vi "Read XML_Extra Checks_Check Tx Channels Default Values Presence.vi"(8 "error in (no error)":errorcluster, 11 "Channels In":T1[](array[typedef])) -> (0 "error out":errorcluster)   [LabVIEW 2016]
doc: "This VI checks that for a given Hardware Channel, all parameters have a unique combination of Parameter settings: Hardware Channel, Label Decimal and Parameter Name. If there are multiple duplicates, the function returns all duplicates."
uses:
  XML_Channel.ctl
  XML_Label.ctl
  XML_Parameter.ctl
  <userlib>/_OpenG.lib/array/array.llb/Filter 1D Array with Scalar (Boolean)__ogtk.vi
panel:
  out "Error Source":string
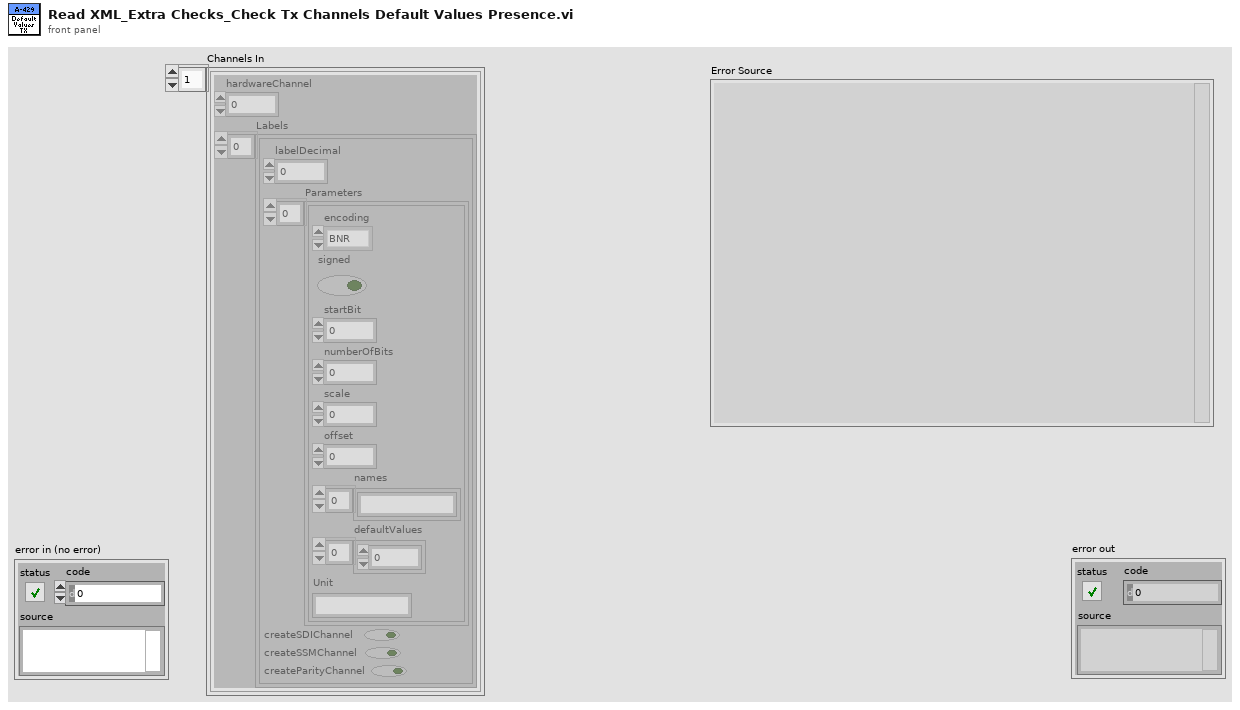
[diagram p1: front panel]
types:
  T1 = typedef "XML_Channel.ctl" = cluster{"hardwareChannel":i32, "Labels":T2[]}
  T2 = typedef "XML_Label.ctl" = cluster{"labelDecimal":i32, "Parameters":T3[], "createSDIChannel":bool, "createSSMChannel":bool, "createParityChannel":bool}
  T3 = typedef "XML_Parameter.ctl" = cluster{"encoding":enum16{"BNR", "BCD", "Discrete"}, "signed":bool, "startBit":i32, "numberOfBits":i32, "scale":dbl, "offset":dbl, "names":string[], "defaultValues":dbl[], "Unit":string}
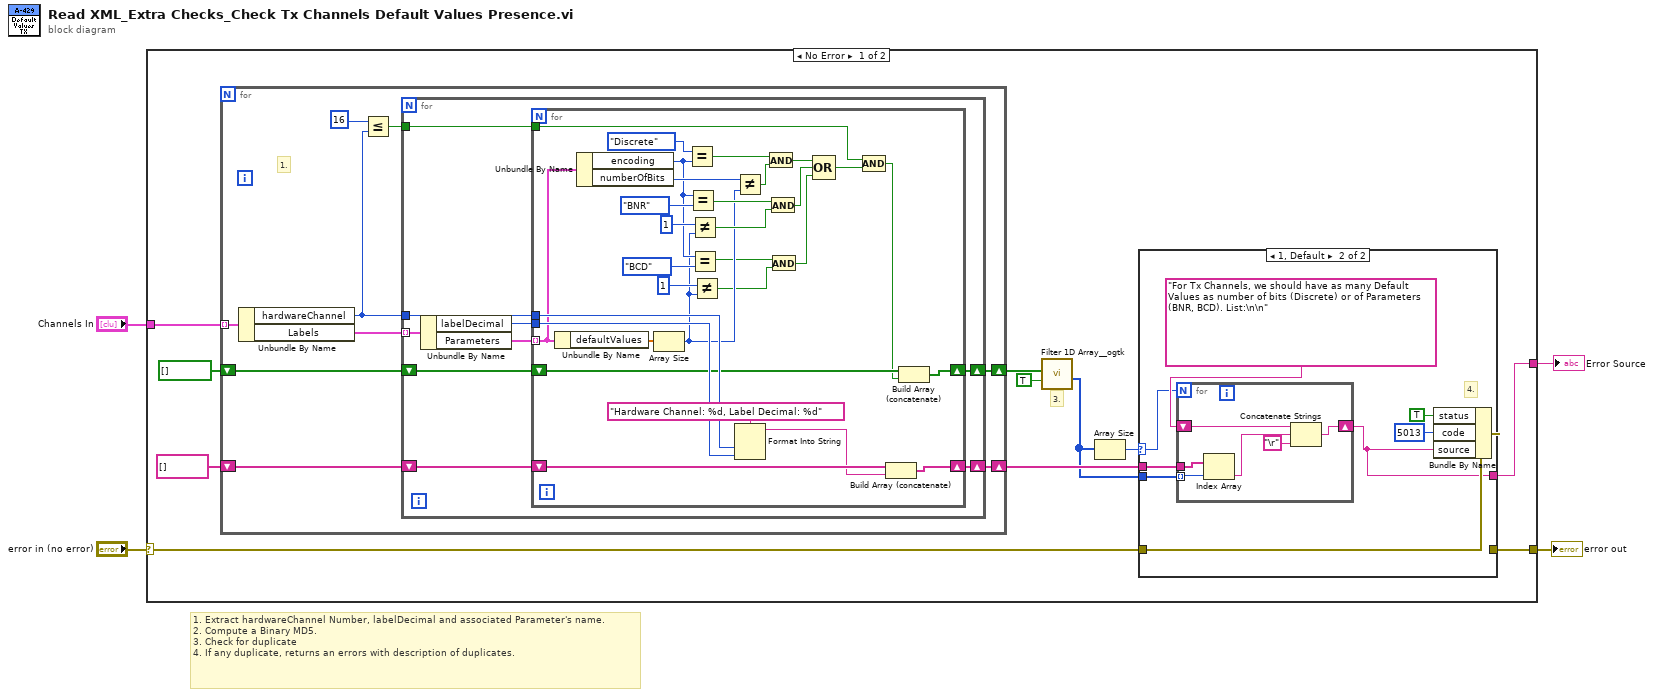
[diagram p0: block diagram]
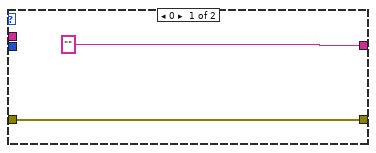
[diagram p2: hidden frame]
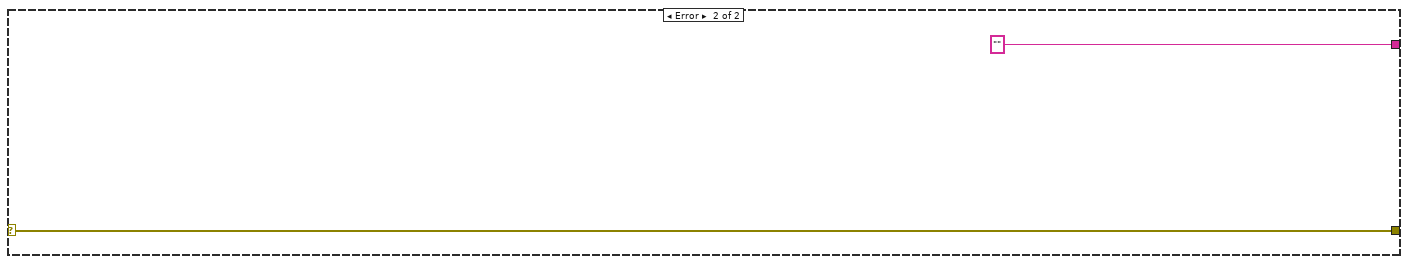
[diagram p3: hidden frame]
diagram:
  # "1. Extract hardwareChannel Number, labelDecimal and associated Parameter's name.\n2. Compute a Binary MD5.\n3. Check for duplicate\n4. If any duplicate, returns an errors with description of duplicates."
  n1 = case shown="No Error" "error in (no error)" {
    selector: "error in (no error)" -> [w14 w82]
    tunnel: [w12 w82] -> w3
    tunnel: "Channels In" -> [w13 _]
    tunnel: [w11 ""] -> w1
    frame No Error {
      # "3."
      n2 = for {
        tunnel: w13 -> [w41] mode=indexing
        shift-right: [w38] -> w8
        shift-left: bool[] [] -> [w39]
        shift-right: [w36] -> w9
        shift-left: string[] [] -> [w37]
        # "1."
        n3 = Unbundle By Name(w41) -> ("hardwareChannel"=w34:i32, "Labels"=w40:T2[])
        n4 = Less Or Equal?(x=16, y=w34) -> (x <= y?=w33:bool)
        n5 = for {
          tunnel: w34 -> [w50]
          tunnel: w40 -> [w49] mode=indexing
          shift-right: [w46] -> w38
          shift-left: w39 -> [w47]
          shift-right: [w43] -> w36
          shift-left: w37 -> [w44]
          tunnel: w33 -> [w42]
          n6 = Unbundle By Name(w49) -> ("labelDecimal"=w48:i32, "Parameters"=w45:T3[])
          n7 = for {
            tunnel: w50 -> [w75]
            tunnel: w48 -> [w80]
            shift-right: [w73] -> w46
            shift-left: w47 -> [w72]
            tunnel: w45 -> [w74] mode=indexing
            shift-right: [w78] -> w43
            shift-left: w44 -> [w79]
            tunnel: w42 -> [w67]
            n8 = Unbundle By Name(w74) -> ("defaultValues"=w71:dbl[])
            n9 = Unbundle By Name(w74) -> ("encoding"=w55:enum16{"BNR", "BCD", "Discrete"}, "numberOfBits"=w70:i32)
            n10 = Array Size(array=w71) -> (size(s)=w54:i32)
            n11 = Equal?(x=enum16{"BNR", "BCD", "Discrete"}."Discrete", y=w55) -> (x = y?=w66:bool)
            n12 = Equal?(x=w55, y=enum16{"BNR", "BCD", "Discrete"}."BNR") -> (x = y?=w61:bool)
            n13 = Not Equal?(x=1, y=w54) -> (x != y?=w59:bool)
            n14 = Equal?(x=w55, y=enum16{"BNR", "BCD", "Discrete"}."BCD") -> (x = y?=w53:bool)
            n15 = Not Equal?(x=1, y=w54) -> (x != y?=w52:bool)
            n16 = Not Equal?(x=w70, y=w54) -> (x != y?=w62:bool)
            n17 = Format Into String(format string="Hardware Channel: %d, Label Decimal: %d", w75, w80) -> (resulting string=w76:string)  [unwired: 2 in, 1 out]
            n18 = And(x=w66, y=w62) -> (x .and. y?=w65:bool)
            n19 = And(x=w61, y=w59) -> (x .and. y?=w58:bool)
            n20 = And(x=w53, y=w52) -> (x .and. y?=w51:bool)
            n21 = Compound Arithmetic op=OR(w65, w58, w51) -> (w64:bool)
            n22 = Compound Arithmetic op=AND(w67, w64) -> (w68:bool)
            n23 = Build Array (concatenate)(w79, w76) -> (w78:string[])
            n24 = Build Array (concatenate)(w72, w68) -> (w73:bool[])
          }
        }
      }
      n25 = call-poly <userlib>:"Filter 1D Array__ogtk.vi"("items to filter"=TRUE, "array"=w8) -> ("filtered item indices"=w7:i32[])  [unwired: 4 in, 1 out]
      n26 = Array Size(array=w7) -> (size(s)=w15:i32)
      n27 = case shown="1, Default" w15 {
        selector: w15 -> [_ w21]
        tunnel: w14 -> [w17 w26]
        tunnel: w7 -> [_ w20]
        tunnel: [w17 w25] -> w12
        tunnel: ["" w19] -> w11
        tunnel: w9 -> [_ w18]
        frame 0 {
        }
        frame 1, Default {
          # "4."
          n28 = for {
            N: w21 -> [_]
            shift-right: [w31] -> w19
            shift-left: "For Tx Channels, we should have as many Default Values as number of bits (Discrete) or of Parameters (BNR, BCD). List:\n\n" -> [w32]
            tunnel: w20 -> [w30] mode=indexing
            tunnel: w18 -> [w28]
            n29 = Index Array(array=w28, index=w30) -> (element=w27:string)
            n30 = Concatenate Strings(w32, w27, "\r") -> (w31:string)
          }
          n31 = Bundle By Name(cluster=w26, "status"=TRUE, "code"=5013, "source"=w19) -> (w25:errorcluster)
        }
      }
    }
    frame Error {
    }
  }
  "error out" <- w3
  "Error Source" <- w1
